vi "Construct RT Seq Top Level.vi"(8 "Error In":errorcluster, 9 "Sequence Cache Path":path, 10 "Log Trigger Name (Aliases/CSVSeqLogTrigger)":string="Aliases/CSVSeqLogTrigger", 11 "CSV File":path) -> (0 "Error Out":errorcluster, 2 "Parameter Defaults":string[][](array[string]), 3 "New RT Seq":path, 5 "1 CSVs Tests":T1)   [LabVIEW 2011]
uses:
  Controls/CSVs Tests Data.ctl
  Controls/Test Column Data.ctl
  NationalInstruments.VeriStand.RealTimeSequenceDefinitionApi
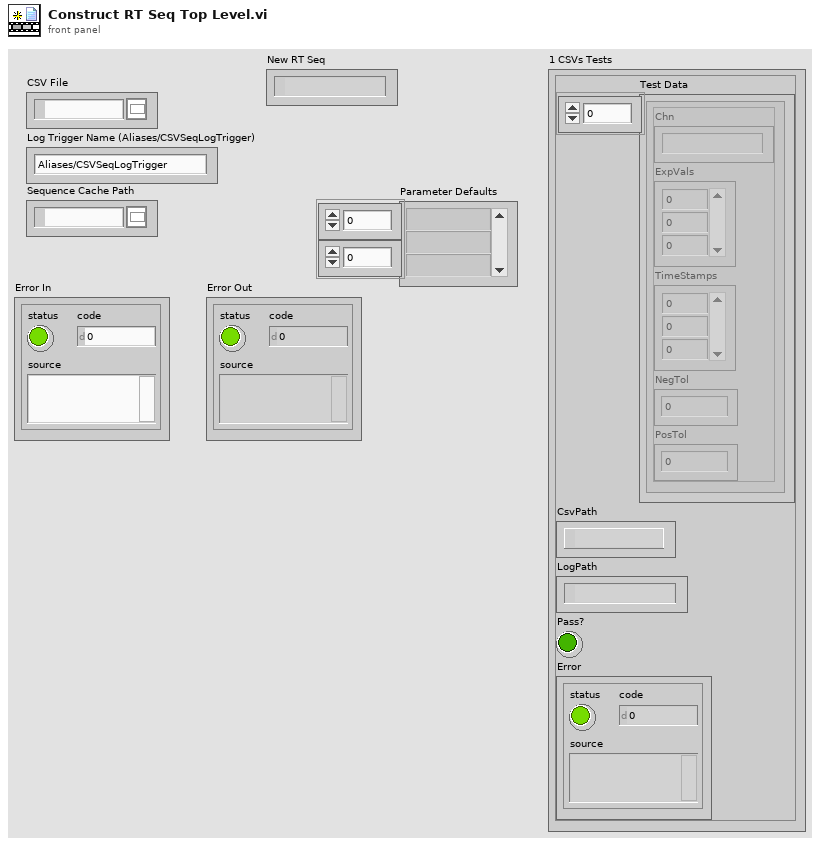
[diagram p1: front panel]
types:
  T1 = typedef "CSVs Tests Data.ctl" = cluster{"Test Data":T2[], "CsvPath":path, "LogPath":path, "Pass?":bool, "Error":errorcluster}
  T2 = typedef "Test Column Data.ctl" = cluster{"Chn":string, "ExpVals":dbl[], "TimeStamps":i64[], "NegTol":dbl, "PosTol":dbl}
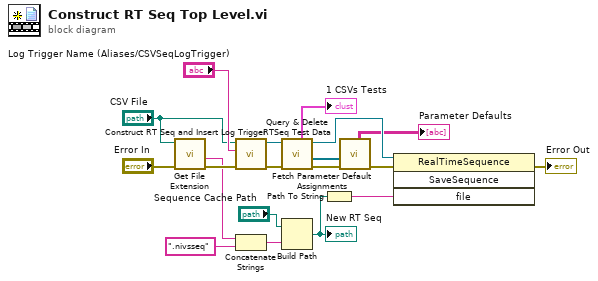
[diagram p0: block diagram]
diagram:
  n1 = call <vilib>:"Get File Extension.vi"("error in (no error)"="Error In", "file"="CSV File") -> ("error out"=w15:errorcluster, "filename without extension"=w14:string)  [unwired: 6 in, 2 out]
  n2 = call "Construct RT Seq and Insert Log Trigger.vi"("Error In"=w15, "Log Trigger Name (Aliases/CSVSeqLogTrigger)"="Log Trigger Name (Aliases/CSVSeqLogTrigger)", "CSV File"="CSV File") -> ("Error Out"=w7:errorcluster, "RT Seq Ref Out"=w8:refnum<k24>)  [unwired: 7 in]
  n3 = Concatenate Strings(w14, ".nivsseq" ("string")) -> (w12:string)
  n4 = call "Query & Delete RTSeq Test Data.vi"("Error In"=w7, "RT Seq Ref In"=w8) -> ("Error Out"=w4:errorcluster, "Parameters"=w2:refnum<k24>[], "RT Seq Ref Out"=w6:refnum<k24>, "1 CSVs Tests"=→"1 CSVs Tests":T1)  [unwired: 6 in]
  n5 = Build Path(base path="Sequence Cache Path", name or relative path=w12) -> (appended path=w10:path)
  "New RT Seq" <- w10
  n6 = Path To String(path=w10) -> (string=w11:string)
  n7 = call "Fetch Parameter Default Assignments.vi"("Error In"=w4, "Parameters"=w2) -> ("Error Out"=w3:errorcluster, "Parameter Defaults"=→"Parameter Defaults":string[][])  [unwired: 8 in]
  n8 = invoke class="RealTimeSequence" method="SaveSequence"(reference=w6, error in=w3, "file"=w11) -> (error out=→"Error Out":errorcluster)  [unwired: 1 in, 3 out]
